vi "Create voltage step array.vi"(0 "Min numb steps":i32=5, 1 "Max voltage jump":dbl, 5 "Setpoint":dbl, 9 "Current/ last  value":dbl, 11 "error in (no error)":errorcluster) -> (8 "Array":dbl[](array[numeric]), 15 "error out":errorcluster)   [LabVIEW 2011]
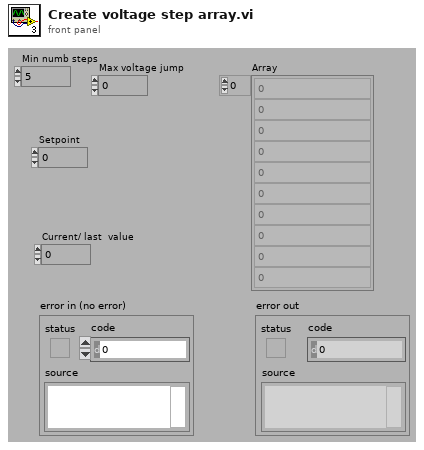
[diagram p1: front panel]
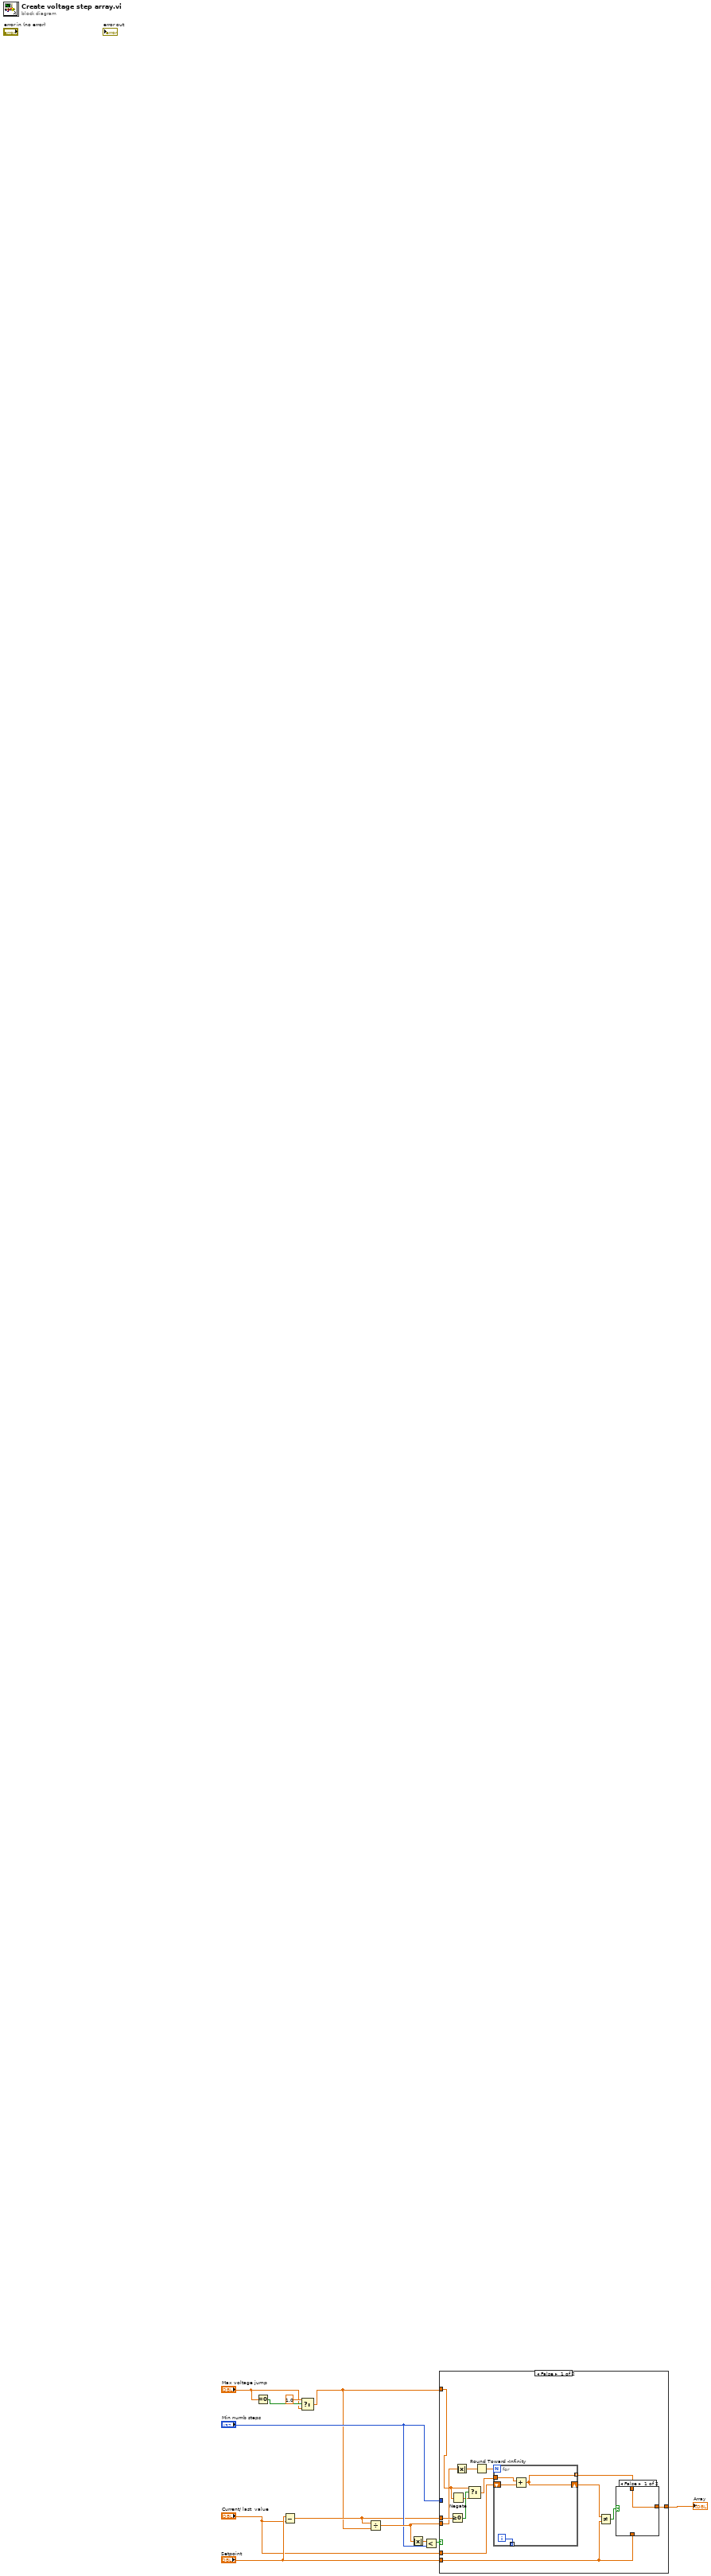
[diagram p0: block diagram]
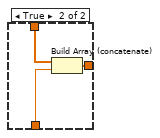
[diagram p2: hidden frame]
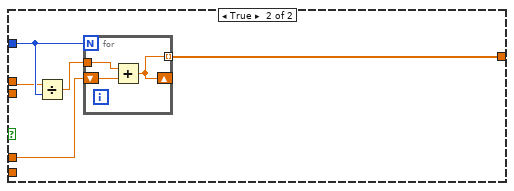
[diagram p3: hidden frame]
diagram:
  n1 = Equal To 0?(x="Max voltage jump") -> (x = 0?=w4:bool)
  n2 = Subtract(x="Setpoint", y="Current/ last  value") -> (x-y=w8:dbl)
  n3 = Select(t=1.0, s=w4, f="Max voltage jump") -> (s? t:f=w1:dbl)
  n4 = Divide(x=w8, y=w1) -> (x/y=w11:dbl)
  n5 = Absolute Value(x=w11) -> (abs(x)=w6:dbl)
  n6 = Less?(x=w6, y="Min numb steps") -> (x < y?=w10:bool)
  n7 = case shown="False" w10 {
    tunnel: w8 -> [w26 w36]
    tunnel: "Setpoint" -> [w15 _]
    tunnel: [w20 w38] -> w12
    tunnel: w11 -> [w23 _]
    tunnel: "Min numb steps" -> [_ w37]
    tunnel: "Current/ last  value" -> [w25 w35]
    tunnel: w1 -> [w18 _]
    frame False {
      n8 = Greater Or Equal To 0?(x=w26) -> (x >= 0?=w19:bool)
      n9 = Negate(x=w18) -> (-x=w17:dbl)
      n10 = Absolute Value(x=w23) -> (abs(x)=w22:dbl)
      n11 = Select(t=w18, s=w19, f=w17) -> (s? t:f=w16:dbl)
      n12 = Round Toward -Infinity(1:w22) -> (0:w21:dbl)
      n13 = for {
        N: w21 -> [_]
        tunnel: w16 -> [w33]
        shift-right: [w32] -> w14
        shift-left: w25 -> [w34]
        tunnel: [w32] -> w24 mode=indexing
        tunnel: [w31] -> _ mode=indexing
        i -> [w31]
        n14 = Add(x=w33, y=w34) -> (x+y=w32:dbl)
      }
      n15 = Not Equal?(x=w14, y=w15) -> (x != y?=w13:bool)
      n16 = case shown="False" w13 {
        tunnel: w24 -> [w27 w30]
        tunnel: [w27 w29] -> w20
        tunnel: w15 -> [_ w28]
        frame False {
        }
        frame True {
          n17 = Build Array (concatenate)(w30, w28) -> (w29:dbl[])
        }
      }
    }
    frame True {
      n18 = Divide(x=w36, y=w37) -> (x/y=w39:dbl)
      n19 = for {
        N: w37 -> [_]
        tunnel: w39 -> [w41]
        shift-right: [w40] -> _
        shift-left: w35 -> [w42]
        tunnel: [w40] -> w38 mode=indexing
        n20 = Add(x=w41, y=w42) -> (x+y=w40:dbl)
      }
    }
  }
  "Array" <- w12
